vi "AssertMultiChannelLoopback.vi"(4 "Tolerance (0.01)":dbl=0.01 format="%#_13g", 6 "Values":dbl[](array[numeric]), 7 "Timeout (1 second)":dbl=1.0 format="%#_13g", 8 "error in (no error)":errorcluster, 9 "Read Channels":string[](array[string]), 10 "Write Channels":string[](array[string]), 11 "VeriStand Test Case in":refnum<class "VeriStandTestCase.lvclass">) -> (0 "error out":errorcluster, 3 "VeriStand Test Case out":refnum<class "VeriStandTestCase.lvclass">)   [LabVIEW 2027, in "VeriStandTestCase.lvclass"]
uses:
  VeriStandTestCase.lvclass
  VeriStandTestCase.lvclass/VeriStandTestCase.ctl
  VeriStandTestUtilities/VeriStandTestUtilities.lvlib
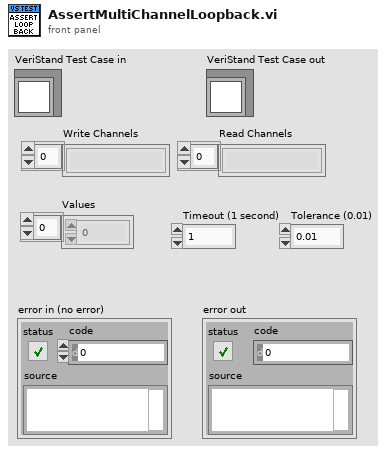
[diagram p1: front panel]
types:
  T1 = typedef "NI_VS Workspace ExecutionAPI.lvlib/WorkspaceAPI.ctl" = refnum<k39>
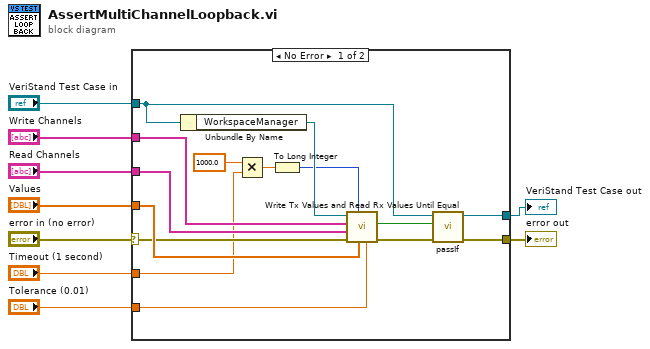
[diagram p0: block diagram]
diagram:
  n1 = case shown="No Error" "error in (no error)" {
    selector: "error in (no error)" -> [w21 w25]
    tunnel: [w24 w25] -> w9
    tunnel: "Read Channels" -> [w17 _]
    tunnel: "Write Channels" -> [w23 _]
    tunnel: "Values" -> [w22 _]
    tunnel: "Timeout (1 second)" -> [w12 _]
    tunnel: "Tolerance (0.01)" -> [w14 _]
    tunnel: "VeriStand Test Case in" -> [w19 w26]
    tunnel: [w20 w26] -> w4
    frame No Error {
      n2 = Unbundle By Name(w19) -> ("WorkspaceManager"=w18:T1)
      n3 = Multiply(x=1000.0, y=w12) -> (x*y=w11:dbl)
      n4 = To Long Integer(number=w11) -> (32bit integer=w10:i32)
      n5 = call "Write Tx Values and Read Rx Values Until Equal.vi"("tolerance (0.01)"=w14, "Tx values"=w22, "timeout (1000 ms)"=w10, "error in"=w21, "Rx aliases"=w17, "Tx aliases"=w23, "workspace manager in"=w18) -> ("error out"=w16:errorcluster, "values equal"=w15:bool)  [unwired: 2 in, 1 out]
      n6 = call-dynamic "passIf.vi"("error in (no error)"=w16, "pass"=w15, "TestCase in"=w19) -> ("error out"=w24:errorcluster, "TestCase out"=w20:refnum<class "VeriStandTestCase.lvclass">)  [unwired: 7 in]
    }
    frame Error {
    }
  }
  "error out" <- w9
  "VeriStand Test Case out" <- w4
